vi "22_09_ex_01.vi"() -> ()   [LabVIEW 2025]
uses:
  <vilib>/numeric/Random Number (Range) U64.vi
  <vilib>/numeric/sub_Random U32.vi
panel:
  out "Array 3":dbl[](array[numeric])
  in  "Array 2":dbl[](array[numeric])
  out "Array":dbl[](array[numeric])
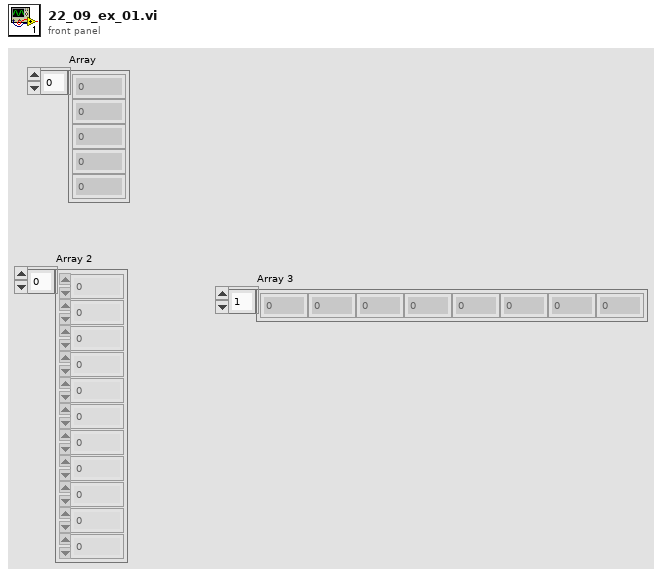
[diagram p1: front panel]
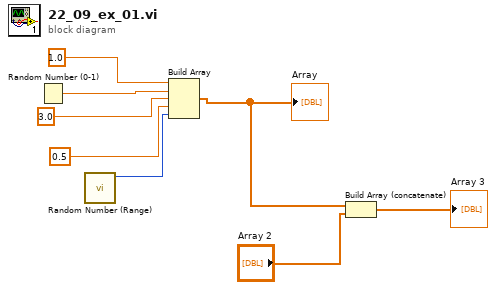
[diagram p0: block diagram]
diagram:
  n1 = Random Number (0-1)() -> (number: 0 to 1=w7:dbl)
  n2 = call-poly <vilib>:"Random Number (Range).vi"() -> ("number"=w5:u64)  [unwired: 11 in]
  n3 = Build Array(1.0 ("element"), w7, 3.0 ("element"), 0.5 ("element"), w5) -> (w1:dbl[])
  "Array" <- w1
  n4 = Build Array (concatenate)(w1, "Array 2") -> (→"Array 3":dbl[])
